vi "setLUT.vi"(2 "Frequency":dbl=1000.0, 3 "Number of entries in LUT":dbl=2048.0, 4 "Count":dbl) -> (0 "Ticks to wait":u32, 1 "Time to wait (s)":dbl)   [LabVIEW 2012]
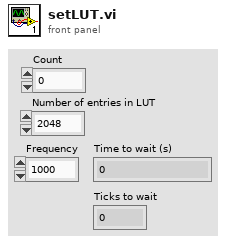
[diagram p1: front panel]
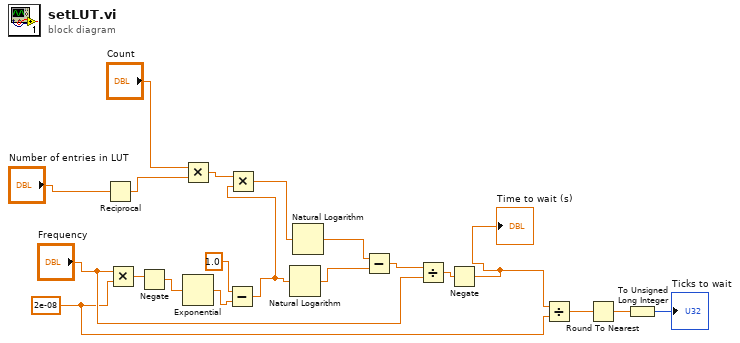
[diagram p0: block diagram]
diagram:
  w17 = 2e-08 ("y")
  n1 = Reciprocal(x="Number of entries in LUT") -> (1/x=w4:dbl)
  n2 = Multiply(x="Frequency", y=w17) -> (x*y=w14:dbl)
  n3 = Negate(x=w14) -> (-x=w13:dbl)
  n4 = Multiply(x="Count", y=w4) -> (x*y=w3:dbl)
  n5 = Exponential(1:w13) -> (0:w11:dbl)
  n6 = Subtract(x=1.0, y=w11) -> (x-y=w2:dbl)
  n7 = Multiply(x=w3, y=w2) -> (x*y=w1:dbl)
  n8 = Natural Logarithm(1:w2) -> (0:w9:dbl)
  n9 = Natural Logarithm(1:w1) -> (0:w10:dbl)
  n10 = Subtract(x=w10, y=w9) -> (x-y=w15:dbl)
  n11 = Divide(x=w15, y="Frequency") -> (x/y=w8:dbl)
  n12 = Negate(x=w8) -> (-x=w7:dbl)
  "Time to wait (s)" <- w7
  n13 = Divide(x=w7, y=w17) -> (x/y=w16:dbl)
  n14 = Round To Nearest(number=w16) -> (nearest integer value=w20:dbl)
  n15 = To Unsigned Long Integer(number=w20) -> (unsigned 32bit integer=→"Ticks to wait":u32)
